vi "DisplayLogic_ScanNextPixel.vi"() -> (16 "ActivePixel":cluster{"h_pixel":i16, "v_pixel":i16})   [LabVIEW 2018]
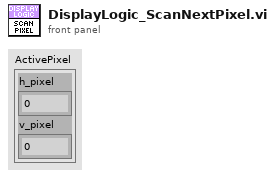
[diagram p1: front panel]
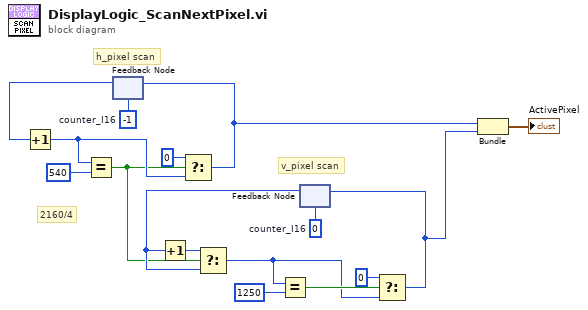
[diagram p0: block diagram]
diagram:
  w9 = i16 0  # counter_I16
  w13 = i16 -1  # counter_I16
  # "2160/4"
  # "v_pixel scan"
  # "h_pixel scan"
  n1 = feedback #1(w13) -> (w12:i16)
  n2 = Increment(x=w12) -> (x+1=w15:i16)
  n3 = Equal?(x=w15, y=i16 540) -> (x = y?=w3:bool)
  n4 = Select(t=i16 0 ("f"), s=w3, f=w15) -> (s? t:f=w1:i16)
  n5 = feedback-in #1(w1) -> ()
  n6 = feedback #2(w9) -> (w5:i16)
  n7 = Increment(x=w5) -> (x+1=w7:i16)
  n8 = Select(t=w7, s=w3, f=w5) -> (s? t:f=w6:i16)
  n9 = Equal?(x=w6, y=i16 1250) -> (x = y?=w8:bool)
  n10 = Select(t=i16 0 ("f"), s=w8, f=w6) -> (s? t:f=w2:i16)
  n11 = feedback-in #2(w2) -> ()
  n12 = Bundle("f"=w1, "counter_I16"=w2) -> (→"ActivePixel":cluster{"f":i16, "counter_I16":i16})  [unwired: 1 in]
